vi "Create ESPEC Temp Tag.vi"(8 "error in (no error)":errorcluster, 11 "CVT Tags to Create":T1) -> (0 "error out":errorcluster, 3 "CVT Tags to Create 2":T1)   [LabVIEW 2021, in "CVT.lvlib"]
uses:
  CVT.lvlib
  Support Libraries/Current Value Table/Type Defs/File Format.ctl
  Support Libraries/Current Value Table/Type Defs/Single Tag.ctl
  Support Libraries/Current Value Table/Type Defs/Data Types.ctl
  Support Libraries/Current Value Table/Type Defs/Tag Grouping set.ctl
  Support Libraries/Current Value Table/Current Value Table.lvlib
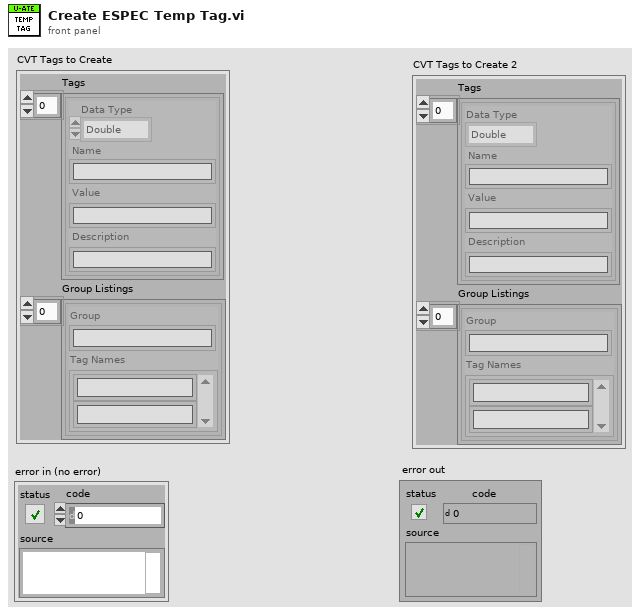
[diagram p1: front panel]
types:
  T1 = typedef "CVT.lvlib/Current Value Table.lvlib/File Format.ctl" = cluster{"Tags":T2[], "Group Listings":T4[]}
  T2 = typedef "CVT.lvlib/Current Value Table.lvlib/Single Tag.ctl" = cluster{"Data Type":T3, "Name":string, "Value":string, "Description":string}
  T3 = typedef "CVT.lvlib/Current Value Table.lvlib/Data Types.ctl" = enum16{"Double", "Single", "I64", "I32", "I16", "I8", "U64", "U32", "U16", "U8", "String", "Boolean", "Array of U8", "Array of U16", "Array of U32", "Array of U64", "Array of I64", "Array of I32", "Array of I16", "Array of I8", "Array of Double", "Array of Single", "Array of Boolean", "Array of String"}
  T4 = typedef "CVT.lvlib/Current Value Table.lvlib/Tag Grouping set.ctl" = cluster{"Group":string, "Tag Names":string[]}
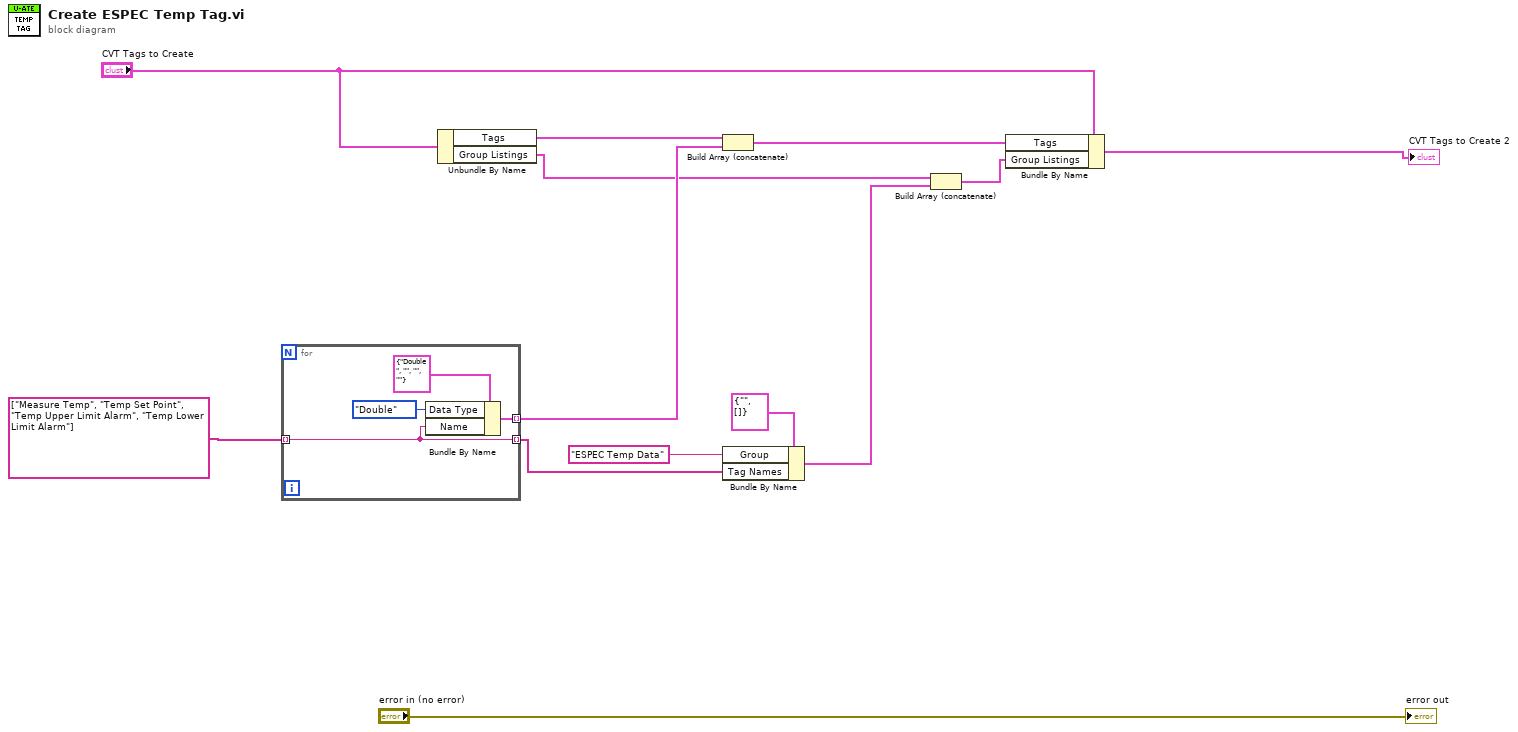
[diagram p0: block diagram]
diagram:
  n1 = for {
    tunnel: string[] ["Measure Temp", "Temp Set Point", "Temp Upper Limit Alarm", "Temp Lower Limit Alarm"] -> [w16] mode=indexing
    tunnel: [w17] -> w8 mode=indexing
    tunnel: [w16] -> w10 mode=indexing
    n2 = Bundle By Name(cluster=T2 {"Data Type"=enum."Double", "Name"="", "Value"="", "Description"=""} ("element"), "Data Type"=Data_Types."Double", "Name"=w16) -> (w17:T2)
  }
  n3 = Unbundle By Name("CVT Tags to Create") -> ("Tags"=w9:T2[], "Group Listings"=w6:T4[])
  n4 = Build Array (concatenate)(w9, w8) -> (w7:T2[])
  n5 = Bundle By Name(cluster=T4 {"Group"="", "Tag Names"=[]} ("Tag Grouping"), "Group"="ESPEC Temp Data", "Tag Names"=w10) -> (w12:T4)
  n6 = Build Array (concatenate)(w6, w12) -> (w5:T4[])
  n7 = Bundle By Name(cluster="CVT Tags to Create", "Tags"=w7, "Group Listings"=w5) -> (→"CVT Tags to Create 2":T1)
  "error out" <- "error in (no error)"
